vi "Read Intrinsic string(SubVI).vi"(8 "error in (no error)":errorcluster, 10 "zmq_socket in":refnum<class "zmq_socket.lvclass">, 11 "Intrinsic Data Cluster TD":T1) -> (0 "error out":errorcluster, 2 "zmq_socket out":refnum<class "zmq_socket.lvclass">, 3 "Intrinsic Data Cluster TD 2":T1)   [LabVIEW 2016]
uses:
  <vilib>/addons/zeromq/zmq_socket.lvclass
  Intrinsic data TD.ctl
panel:
  out "data":string
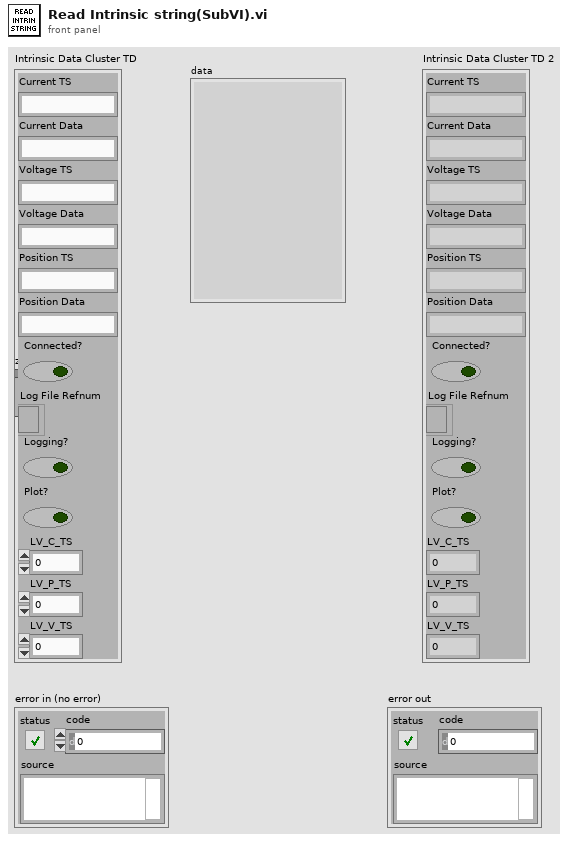
[diagram p1: front panel]
types:
  T1 = typedef "Intrinsic data TD.ctl" = cluster{"Current TS":string, "Current Data":string, "Voltage TS":string, "Voltage Data":string, "Position TS":string, "Position Data":string, "Connected?":bool, "Log File Refnum":refnum<file>, "Logging?":bool, "Plot?":bool, "LV_C_TS":dbl, "LV_P_TS":dbl, "LV_V_TS":dbl}
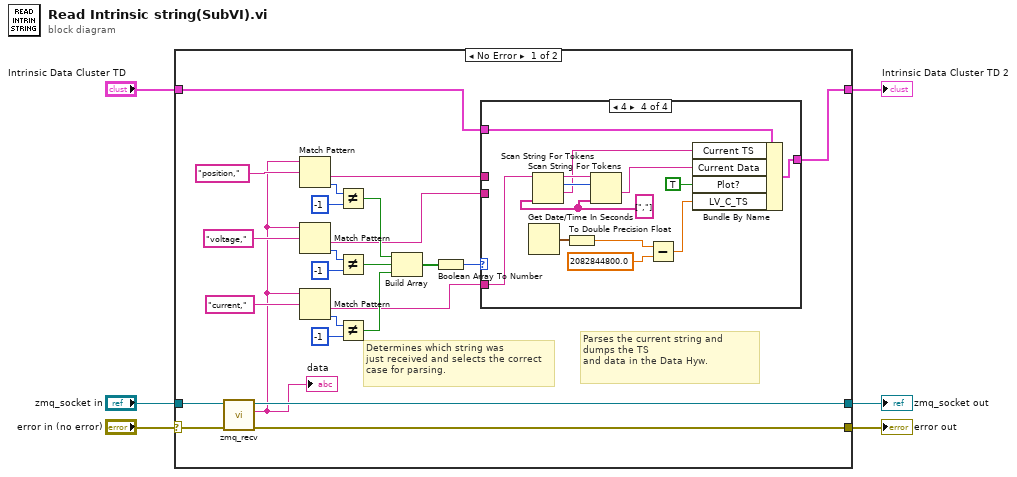
[diagram p0: block diagram]
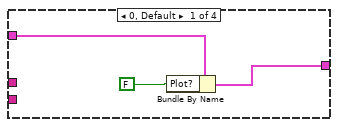
[diagram p2: hidden frame]
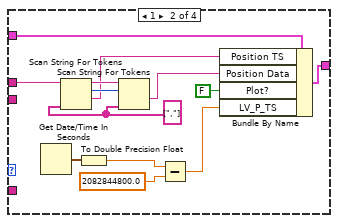
[diagram p3: hidden frame]
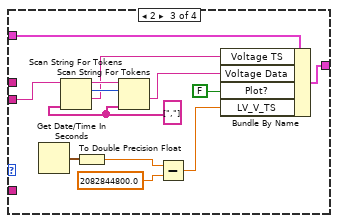
[diagram p4: hidden frame]
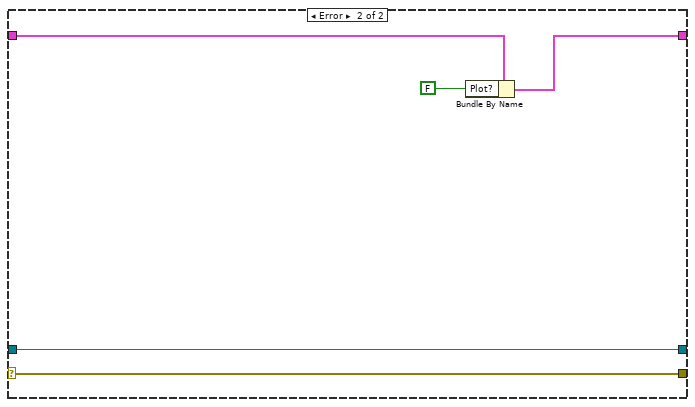
[diagram p5: hidden frame]
diagram:
  n1 = case shown="No Error" "error in (no error)" {
    selector: "error in (no error)" -> [w26 w77]
    tunnel: [w27 w77] -> w6
    tunnel: [w25 w76] -> w4
    tunnel: "zmq_socket in" -> [w24 w76]
    tunnel: [w14 w74] -> w1
    tunnel: "Intrinsic Data Cluster TD" -> [w15 w75]
    frame No Error {
      # "Determines which string was \njust received and selects the correct\ncase for parsing."
      # "Parses the current string and dumps the TS\nand data in the Data Hyw."
      n2 = call <vilib>:"zmq_recv.vi"("error in"=w26, "socket in"=w24) -> ("error out"=w27:errorcluster, "data"=w17:string, "socket out"=w25:refnum<class "zmq_socket.lvclass">)  [unwired: 3 in, 2 out]
      "data" <- w17
      n3 = Match Pattern(string=w17, regular expression="position,") -> (after substring=w16:string, offset past match=w20:i32)  [unwired: 1 in, 2 out]
      n4 = Match Pattern(string=w17, regular expression="voltage,") -> (after substring=w8:string, offset past match=w21:i32)  [unwired: 1 in, 2 out]
      n5 = Match Pattern(string=w17, regular expression="current,") -> (after substring=w7:string, offset past match=w30:i32)  [unwired: 1 in, 2 out]
      n6 = Not Equal?(x=w20, y=-1) -> (x != y?=w12:bool)
      n7 = Not Equal?(x=w21, y=-1) -> (x != y?=w11:bool)
      n8 = Not Equal?(x=w30, y=-1) -> (x != y?=w10:bool)
      n9 = Build Array(w12, w11, w10) -> (w13:bool[])
      n10 = Boolean Array To Number(Boolean array=w13) -> (number=w9:u32)
      n11 = case shown="4" w9 {
        tunnel: w16 -> [_ w46 _ _]
        tunnel: w15 -> [w33 w42 w56 w69]
        tunnel: [w32 w39 w53 w66] -> w14
        tunnel: w8 -> [_ _ w52 _]
        tunnel: w7 -> [_ _ _ w65]
        frame 0, Default {
          n12 = Bundle By Name(cluster=w33, "Plot?"=FALSE) -> (w32:T1)
        }
        frame 1 {
          w45 = string[] [","]
          n13 = Get Date/Time In Seconds() -> (seconds since 1Jan1904=w37:timestamp)
          n14 = Scan String For Tokens(6:w45, 9:w46) -> (1:w41:string, 2:w43:i32, 3:w44:string)  [unwired: 4 in, 1 out]
          n15 = To Double Precision Float(number=w37) -> (double precision float=w36:dbl)
          n16 = Scan String For Tokens(6:w45, 8:w43, 9:w44) -> (1:w40:string)  [unwired: 3 in, 3 out]
          n17 = Subtract(x=w36, y=2082844800.0 ("Epoch Delta (s)")) -> (x-y=w34:dbl)
          n18 = Bundle By Name(cluster=w42, "Position TS"=w41, "Position Data"=w40, "Plot?"=FALSE, "LV_P_TS"=w34) -> (w39:T1)
        }
        frame 2 {
          w59 = string[] [","]
          n19 = Get Date/Time In Seconds() -> (seconds since 1Jan1904=w50:timestamp)
          n20 = Scan String For Tokens(6:w59, 9:w52) -> (1:w55:string, 2:w57:i32, 3:w58:string)  [unwired: 4 in, 1 out]
          n21 = To Double Precision Float(number=w50) -> (double precision float=w49:dbl)
          n22 = Scan String For Tokens(6:w59, 8:w57, 9:w58) -> (1:w54:string)  [unwired: 3 in, 3 out]
          n23 = Subtract(x=w49, y=2082844800.0 ("Epoch Delta (s)")) -> (x-y=w47:dbl)
          n24 = Bundle By Name(cluster=w56, "Voltage TS"=w55, "Voltage Data"=w54, "Plot?"=FALSE, "LV_V_TS"=w47) -> (w53:T1)
        }
        frame 4 {
          w72 = string[] [","]
          n25 = Get Date/Time In Seconds() -> (seconds since 1Jan1904=w63:timestamp)
          n26 = Scan String For Tokens(6:w72, 9:w65) -> (1:w68:string, 2:w70:i32, 3:w71:string)  [unwired: 4 in, 1 out]
          n27 = To Double Precision Float(number=w63) -> (double precision float=w62:dbl)
          n28 = Scan String For Tokens(6:w72, 8:w70, 9:w71) -> (1:w67:string)  [unwired: 3 in, 3 out]
          n29 = Subtract(x=w62, y=2082844800.0 ("Epoch Delta (s)")) -> (x-y=w60:dbl)
          n30 = Bundle By Name(cluster=w69, "Current TS"=w68, "Current Data"=w67, "Plot?"=TRUE, "LV_C_TS"=w60) -> (w66:T1)
        }
      }
    }
    frame Error {
      n31 = Bundle By Name(cluster=w75, "Plot?"=FALSE) -> (w74:T1)
    }
  }
  "error out" <- w6
  "zmq_socket out" <- w4
  "Intrinsic Data Cluster TD 2" <- w1
